vi "Math_2_Term_API_Hierarchy.vi"   [LabVIEW 2021]
uses:
  Support/Add/DBL/Add_DBL.lvclass
  Support/Subtract/DBL/Subtract_DBL.lvclass
  Support/Function/Two Terminal/SGL/AbsFunc_Two Term_SGL.lvclass
  Support/Function/Two Terminal/DBL/AbsFunc_Two Term_DBL.lvclass
  Support/Function/Two Terminal/EXT/AbsFunc_Two Term_EXT.lvclass
  Support/Function/Two Terminal/Cmplx SGL/AbsFunc_Two Term_Complex SGL.lvclass
  Support/Function/Two Terminal/Cmplx DBL/AbsFunc_Two Term_Complex DBL.lvclass
  Support/Function/Two Terminal/Cmplx EXT/AbsFunc_Two Term_Complex EXT.lvclass
  Support/Function/Two Terminal/I8/AbsFunc_Two Term_I8.lvclass
  Support/Function/Two Terminal/I16/AbsFunc_Two Term_I16.lvclass
  Support/Function/Two Terminal/I32/AbsFunc_Two Term_I32.lvclass
  Support/Function/Two Terminal/I64/AbsFunc_Two Term_I64.lvclass
  Support/Function/Two Terminal/U8/AbsFunc_Two Term_U8.lvclass
  Support/Function/Two Terminal/U16/AbsFunc_Two Term_U16.lvclass
  Support/Function/Two Terminal/U32/AbsFunc_Two Term_U32.lvclass
  Support/Function/Two Terminal/U64/AbsFunc_Two Term_U64.lvclass
  Support/Function/Two Terminal/WFM_Numeric/AbsFunc_Two Term_WFM_Numeric.lvclass
  Support/Function/Two Terminal/Time/AbsFunc_Two Term_Time.lvclass
  Support/Add/SGL/Add_SGL.lvclass
  Support/Add/EXT/Add_EXT.lvclass
  Support/Add/CPLX_SGL/Add_CPLX_SGL.lvclass
  Support/Add/CPLX_DBL/Add_CPLX_DBL.lvclass
  Support/Add/CPLX_EXT/Add_CPLX_EXT.lvclass
  Support/Add/I8/Add_I8.lvclass
  Support/Add/I16/Add_I16.lvclass
  Support/Add/I32/Add_I32.lvclass
  Support/Add/I64/Add_I64.lvclass
  Support/Add/U8/Add_U8.lvclass
  Support/Add/U16/Add_U16.lvclass
  Support/Add/U32/Add_U32.lvclass
  Support/Add/U64/Add_U64.lvclass
  Support/Add/Time/Add_Time.lvclass
  Support/Add/WFM_Numeric/Add_WFM_Numeric.lvclass
  Support/Subtract/SGL/Subtract_SGL.lvclass
  Support/Subtract/EXT/Subtract_EXT.lvclass
  Support/Subtract/CPLX_SGL/Subtract_CPLX_SGL.lvclass
  Support/Subtract/CPLX_DBL/Subtract_CPLX_DBL.lvclass
  Support/Subtract/CPLX_EXT/Subtract_CPLX_EXT.lvclass
  Support/Subtract/I8/Subtract_I8.lvclass
  Support/Subtract/I16/Subtract_I16.lvclass
  Support/Subtract/I32/Subtract_I32.lvclass
  Support/Subtract/I64/Subtract_I64.lvclass
  Support/Subtract/U8/Subtract_U8.lvclass
  Support/Subtract/U16/Subtract_U16.lvclass
  Support/Subtract/U32/Subtract_U32.lvclass
  Support/Subtract/U64/Subtract_U64.lvclass
  Support/Subtract/Time/Subtract_Time.lvclass
  Support/Multiply/DBL/Multiply_DBL.lvclass
  Support/Subtract/WFM_Numeric/Subtract_WFM_Numeric.lvclass
  Support/Multiply/SGL/Multiply_SGL.lvclass
  Support/Multiply/EXT/Multiply_EXT.lvclass
  Support/Multiply/CPLX_SGL/Multiply_CPLX_SGL.lvclass
  Support/Multiply/CPLX_DBL/Multiply_CPLX_DBL.lvclass
  Support/Multiply/CPLX_EXT/Multiply_CPLX_EXT.lvclass
  Support/Multiply/I8/Multiply_I8.lvclass
  Support/Multiply/I16/Multiply_I16.lvclass
  Support/Multiply/I32/Multiply_I32.lvclass
  Support/Multiply/I64/Multiply_I64.lvclass
  Support/Multiply/U8/Multiply_U8.lvclass
  Support/Multiply/U16/Multiply_U16.lvclass
  Support/Multiply/U32/Multiply_U32.lvclass
  Support/Multiply/U64/Multiply_U64.lvclass
  Support/Multiply/WFM_Numeric/Multiply_WFM_Numeric.lvclass
  Support/Divide/SGL/Divide_SGL.lvclass
  Support/Divide/DBL/Divide_DBL.lvclass
  Support/Divide/EXT/Divide_EXT.lvclass
  Support/Divide/CPLX_DBL/Divide_CPLX_DBL.lvclass
  Support/Divide/CPLX_EXT/Divide_CPLX_EXT.lvclass
  Support/Divide/CPLX_SGL/Divide_CPLX_SGL.lvclass
  Support/Divide/WFM_Numeric/Divide_WFM_Numeric.lvclass
  Support/Subtract/Time-Time/Subtract_Time-Time.lvclass
  Abs_Types/Double Float/Abs_Double Float.lvclass
  Support/Divide/INT/Divide_INT.lvclass
panel:
  # "SEE DIAGRAM\nFOR Hierarchy"
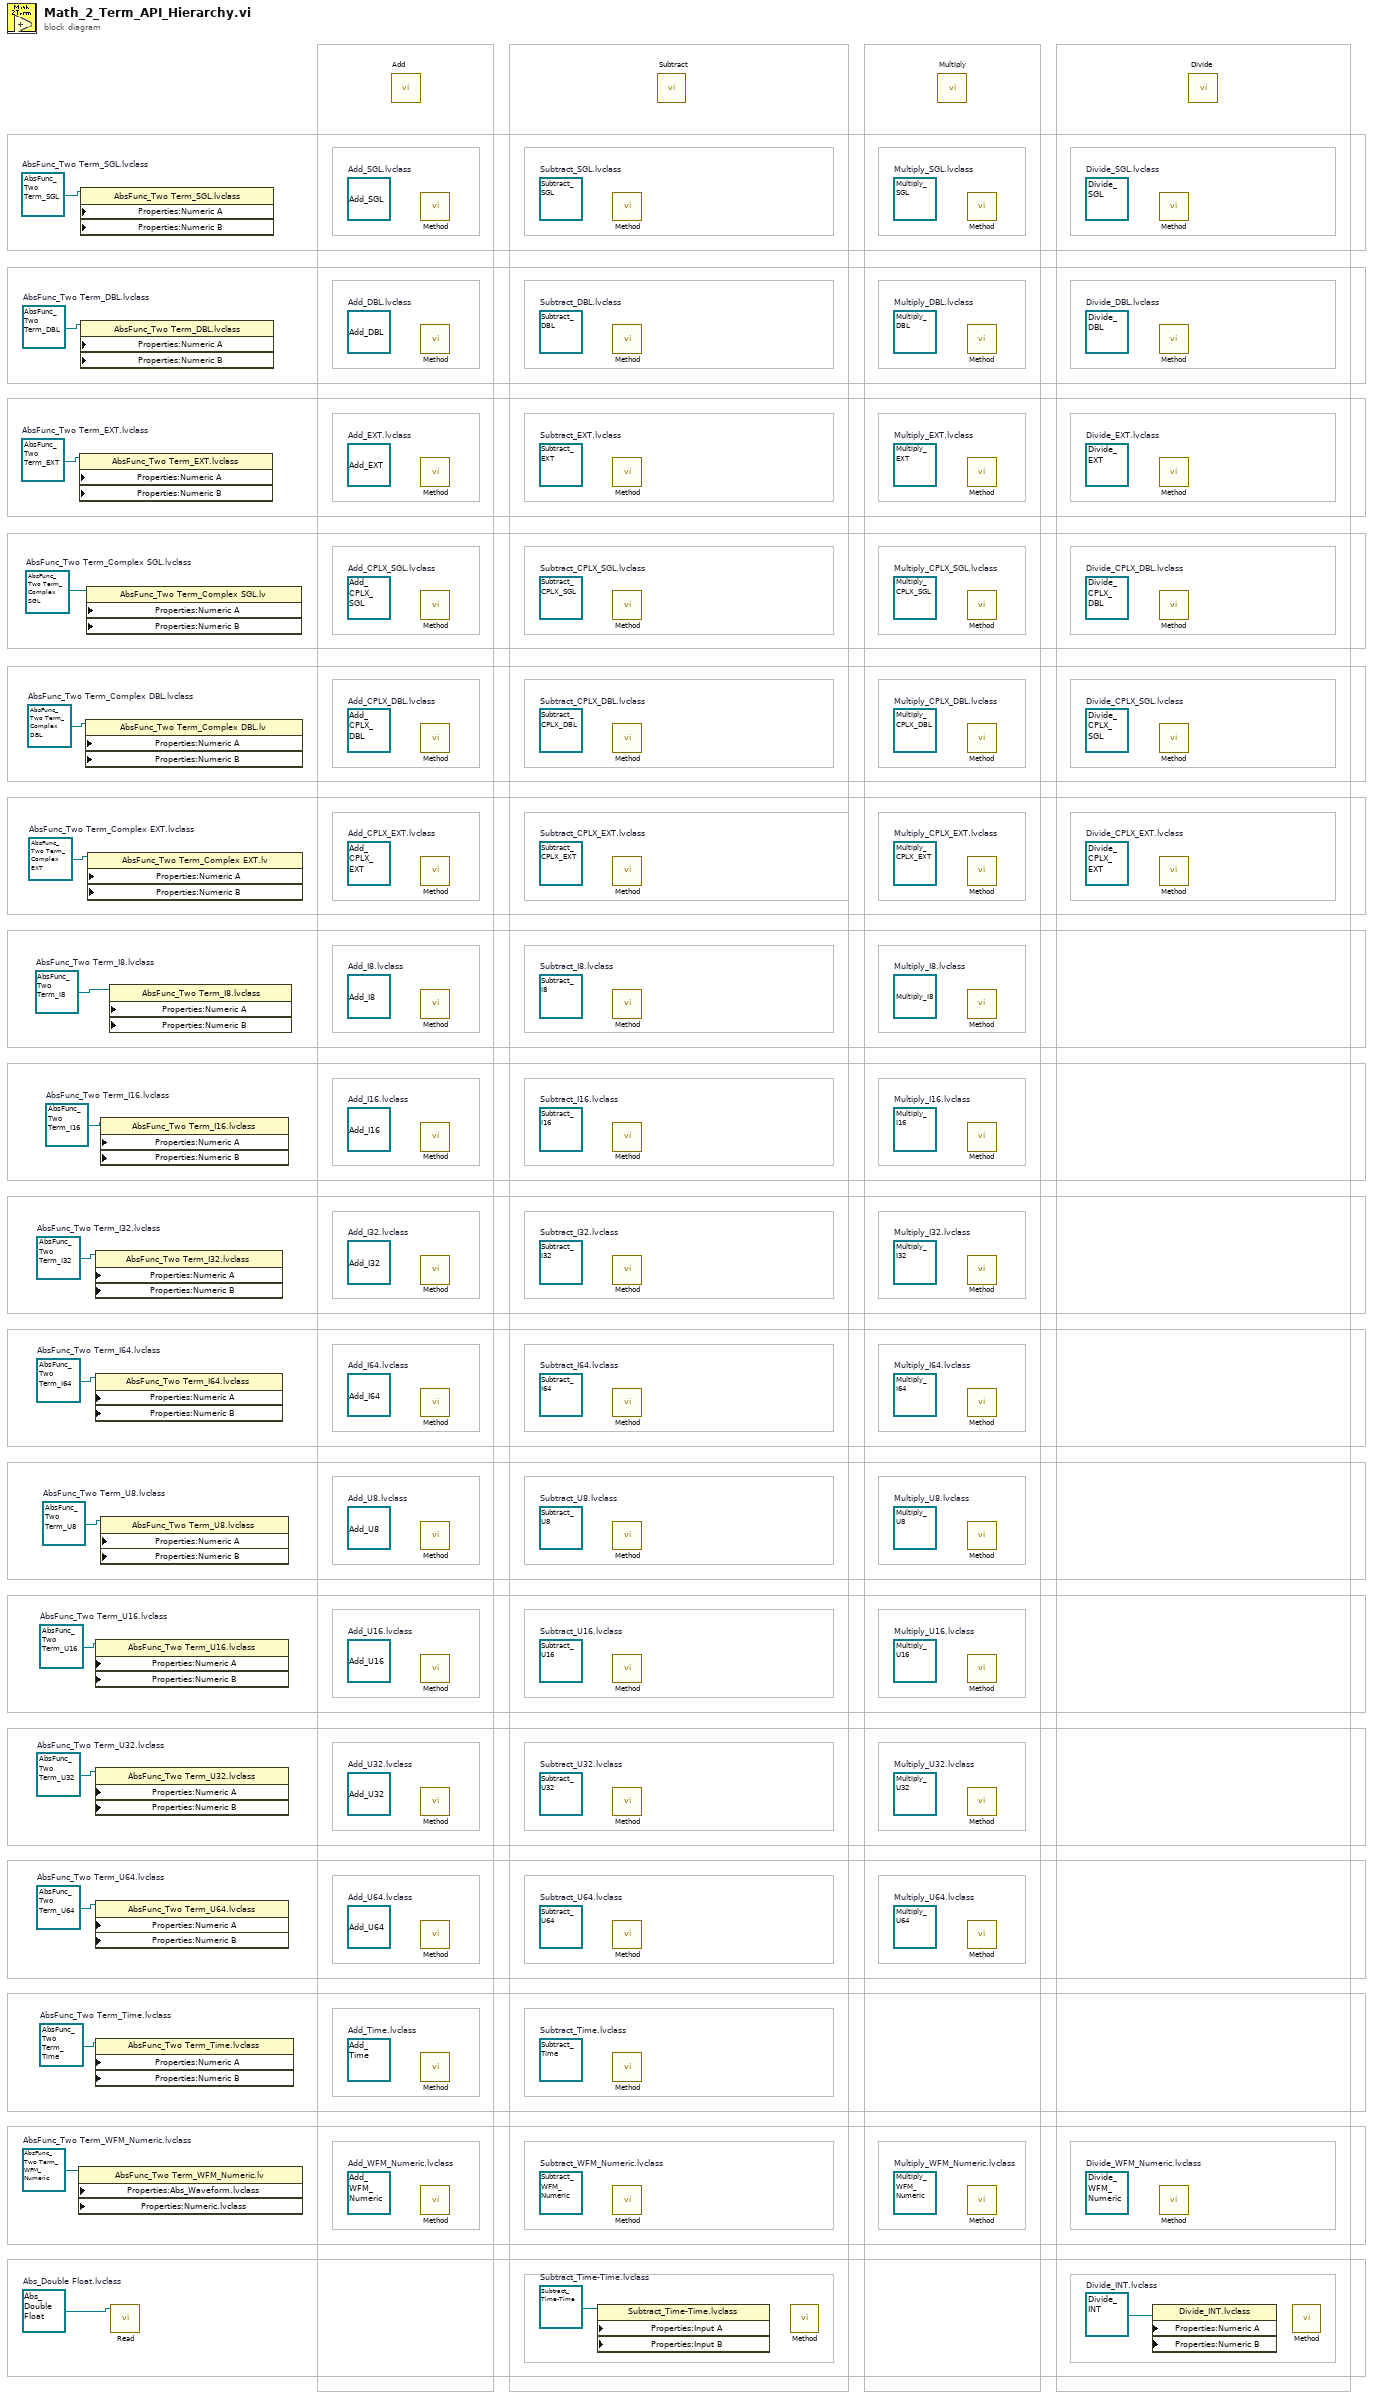
[diagram p0: block diagram]
diagram:
  w1 = refnum<class "Divide_INT.lvclass"> refnum  # Divide_INT.lvclass
  w2 = refnum<class "Abs_Double Float.lvclass"> refnum  # Abs_Double Float.lvclass
  w3 = refnum<class "Subtract_Time-Time.lvclass"> refnum  # Subtract_Time-Time.lvclass
  (unwired) refnum<class "Divide_WFM_Numeric.lvclass"> refnum  # Divide_WFM_Numeric.lvclass
  (unwired) refnum<class "Divide_CPLX_SGL.lvclass"> refnum  # Divide_CPLX_SGL.lvclass
  (unwired) refnum<class "Divide_CPLX_EXT.lvclass"> refnum  # Divide_CPLX_EXT.lvclass
  (unwired) refnum<class "Divide_CPLX_DBL.lvclass"> refnum  # Divide_CPLX_DBL.lvclass
  (unwired) refnum<class "Divide_EXT.lvclass"> refnum  # Divide_EXT.lvclass
  (unwired) refnum<class "Divide_DBL.lvclass"> refnum  # Divide_DBL.lvclass
  (unwired) refnum<class "Divide_SGL.lvclass"> refnum  # Divide_SGL.lvclass
  (unwired) refnum<class "Multiply_WFM_Numeric.lvclass"> refnum  # Multiply_WFM_Numeric.lvclass
  (unwired) refnum<class "Multiply_U64.lvclass"> refnum  # Multiply_U64.lvclass
  (unwired) refnum<class "Multiply_U32.lvclass"> refnum  # Multiply_U32.lvclass
  (unwired) refnum<class "Multiply_U16.lvclass"> refnum  # Multiply_U16.lvclass
  (unwired) refnum<class "Multiply_U8.lvclass"> refnum  # Multiply_U8.lvclass
  (unwired) refnum<class "Multiply_I64.lvclass"> refnum  # Multiply_I64.lvclass
  (unwired) refnum<class "Multiply_I32.lvclass"> refnum  # Multiply_I32.lvclass
  (unwired) refnum<class "Multiply_I16.lvclass"> refnum  # Multiply_I16.lvclass
  (unwired) refnum<class "Multiply_I8.lvclass"> refnum  # Multiply_I8.lvclass
  (unwired) refnum<class "Multiply_CPLX_EXT.lvclass"> refnum  # Multiply_CPLX_EXT.lvclass
  (unwired) refnum<class "Multiply_CPLX_DBL.lvclass"> refnum  # Multiply_CPLX_DBL.lvclass
  (unwired) refnum<class "Multiply_CPLX_SGL.lvclass"> refnum  # Multiply_CPLX_SGL.lvclass
  (unwired) refnum<class "Multiply_EXT.lvclass"> refnum  # Multiply_EXT.lvclass
  (unwired) refnum<class "Multiply_DBL.lvclass"> refnum  # Multiply_DBL.lvclass
  (unwired) refnum<class "Multiply_SGL.lvclass"> refnum  # Multiply_SGL.lvclass
  (unwired) refnum<class "Subtract_WFM_Numeric.lvclass"> refnum  # Subtract_WFM_Numeric.lvclass
  (unwired) refnum<class "Subtract_Time.lvclass"> refnum  # Subtract_Time.lvclass
  (unwired) refnum<class "Subtract_U64.lvclass"> refnum  # Subtract_U64.lvclass
  (unwired) refnum<class "Subtract_U32.lvclass"> refnum  # Subtract_U32.lvclass
  (unwired) refnum<class "Subtract_U16.lvclass"> refnum  # Subtract_U16.lvclass
  (unwired) refnum<class "Subtract_U8.lvclass"> refnum  # Subtract_U8.lvclass
  (unwired) refnum<class "Subtract_I64.lvclass"> refnum  # Subtract_I64.lvclass
  (unwired) refnum<class "Subtract_I32.lvclass"> refnum  # Subtract_I32.lvclass
  (unwired) refnum<class "Subtract_I16.lvclass"> refnum  # Subtract_I16.lvclass
  (unwired) refnum<class "Subtract_I8.lvclass"> refnum  # Subtract_I8.lvclass
  (unwired) refnum<class "Subtract_CPLX_EXT.lvclass"> refnum  # Subtract_CPLX_EXT.lvclass
  (unwired) refnum<class "Subtract_CPLX_DBL.lvclass"> refnum  # Subtract_CPLX_DBL.lvclass
  (unwired) refnum<class "Subtract_CPLX_SGL.lvclass"> refnum  # Subtract_CPLX_SGL.lvclass
  (unwired) refnum<class "Subtract_EXT.lvclass"> refnum  # Subtract_EXT.lvclass
  (unwired) refnum<class "Subtract_DBL.lvclass"> refnum  # Subtract_DBL.lvclass
  (unwired) refnum<class "Subtract_SGL.lvclass"> refnum  # Subtract_SGL.lvclass
  (unwired) refnum<class "Add_WFM_Numeric.lvclass"> refnum  # Add_WFM_Numeric.lvclass
  (unwired) refnum<class "Add_Time.lvclass"> refnum  # Add_Time.lvclass
  (unwired) refnum<class "Add_U64.lvclass"> refnum  # Add_U64.lvclass
  (unwired) refnum<class "Add_U32.lvclass"> refnum  # Add_U32.lvclass
  (unwired) refnum<class "Add_U16.lvclass"> refnum  # Add_U16.lvclass
  (unwired) refnum<class "Add_U8.lvclass"> refnum  # Add_U8.lvclass
  (unwired) refnum<class "Add_I64.lvclass"> refnum  # Add_I64.lvclass
  (unwired) refnum<class "Add_I32.lvclass"> refnum  # Add_I32.lvclass
  (unwired) refnum<class "Add_I16.lvclass"> refnum  # Add_I16.lvclass
  (unwired) refnum<class "Add_I8.lvclass"> refnum  # Add_I8.lvclass
  (unwired) refnum<class "Add_CPLX_EXT.lvclass"> refnum  # Add_CPLX_EXT.lvclass
  (unwired) refnum<class "Add_CPLX_DBL.lvclass"> refnum  # Add_CPLX_DBL.lvclass
  (unwired) refnum<class "Add_CPLX_SGL.lvclass"> refnum  # Add_CPLX_SGL.lvclass
  (unwired) refnum<class "Add_EXT.lvclass"> refnum  # Add_EXT.lvclass
  (unwired) refnum<class "Add_SGL.lvclass"> refnum  # Add_SGL.lvclass
  (unwired) refnum<class "Add_DBL.lvclass"> refnum  # Add_DBL.lvclass
  w4 = refnum<class "AbsFunc_Two Term_Time.lvclass"> refnum  # AbsFunc_Two Term_Time.lvclass
  w5 = refnum<class "AbsFunc_Two Term_WFM_Numeric.lvclass"> refnum  # AbsFunc_Two Term_WFM_Numeric.lvclass
  w6 = refnum<class "AbsFunc_Two Term_U64.lvclass"> refnum  # AbsFunc_Two Term_U64.lvclass
  w7 = refnum<class "AbsFunc_Two Term_U32.lvclass"> refnum  # AbsFunc_Two Term_U32.lvclass
  w8 = refnum<class "AbsFunc_Two Term_U16.lvclass"> refnum  # AbsFunc_Two Term_U16.lvclass
  w9 = refnum<class "AbsFunc_Two Term_U8.lvclass"> refnum  # AbsFunc_Two Term_U8.lvclass
  w10 = refnum<class "AbsFunc_Two Term_I64.lvclass"> refnum  # AbsFunc_Two Term_I64.lvclass
  w11 = refnum<class "AbsFunc_Two Term_I32.lvclass"> refnum  # AbsFunc_Two Term_I32.lvclass
  w12 = refnum<class "AbsFunc_Two Term_I16.lvclass"> refnum  # AbsFunc_Two Term_I16.lvclass
  w13 = refnum<class "AbsFunc_Two Term_I8.lvclass"> refnum  # AbsFunc_Two Term_I8.lvclass
  w14 = refnum<class "AbsFunc_Two Term_Complex EXT.lvclass"> refnum  # AbsFunc_Two Term_Complex EXT.lvclass
  w15 = refnum<class "AbsFunc_Two Term_Complex DBL.lvclass"> refnum  # AbsFunc_Two Term_Complex DBL.lvclass
  w16 = refnum<class "AbsFunc_Two Term_Complex SGL.lvclass"> refnum  # AbsFunc_Two Term_Complex SGL.lvclass
  w17 = refnum<class "AbsFunc_Two Term_EXT.lvclass"> refnum  # AbsFunc_Two Term_EXT.lvclass
  w18 = refnum<class "AbsFunc_Two Term_DBL.lvclass"> refnum  # AbsFunc_Two Term_DBL.lvclass
  w19 = refnum<class "AbsFunc_Two Term_SGL.lvclass"> refnum  # AbsFunc_Two Term_SGL.lvclass
  n1 = property class="AbsFunc_Two Term_WFM_Numeric.lv" props=["Properties:Abs_Waveform.lvclass", "Properties:Numeric.lvclass"](reference=w5) -> ()  [unwired: 3 in, 2 out]
  n2 = property class="AbsFunc_Two Term_EXT.lvclass" props=["Properties:Numeric A", "Properties:Numeric B"](reference=w17) -> ()  [unwired: 3 in, 2 out]
  n3 = property class="AbsFunc_Two Term_SGL.lvclass" props=["Properties:Numeric A", "Properties:Numeric B"](reference=w19) -> ()  [unwired: 3 in, 2 out]
  n4 = property class="AbsFunc_Two Term_DBL.lvclass" props=["Properties:Numeric A", "Properties:Numeric B"](reference=w18) -> ()  [unwired: 3 in, 2 out]
  n5 = property class="AbsFunc_Two Term_Complex DBL.lv" props=["Properties:Numeric A", "Properties:Numeric B"](reference=w15) -> ()  [unwired: 3 in, 2 out]
  n6 = property class="AbsFunc_Two Term_Complex SGL.lv" props=["Properties:Numeric A", "Properties:Numeric B"](reference=w16) -> ()  [unwired: 3 in, 2 out]
  n7 = property class="AbsFunc_Two Term_Complex EXT.lv" props=["Properties:Numeric A", "Properties:Numeric B"](reference=w14) -> ()  [unwired: 3 in, 2 out]
  n8 = property class="AbsFunc_Two Term_I32.lvclass" props=["Properties:Numeric A", "Properties:Numeric B"](reference=w11) -> ()  [unwired: 3 in, 2 out]
  n9 = property class="AbsFunc_Two Term_I64.lvclass" props=["Properties:Numeric A", "Properties:Numeric B"](reference=w10) -> ()  [unwired: 3 in, 2 out]
  n10 = property class="AbsFunc_Two Term_U16.lvclass" props=["Properties:Numeric A", "Properties:Numeric B"](reference=w8) -> ()  [unwired: 3 in, 2 out]
  n11 = property class="AbsFunc_Two Term_U32.lvclass" props=["Properties:Numeric A", "Properties:Numeric B"](reference=w7) -> ()  [unwired: 3 in, 2 out]
  n12 = property class="AbsFunc_Two Term_U64.lvclass" props=["Properties:Numeric A", "Properties:Numeric B"](reference=w6) -> ()  [unwired: 3 in, 2 out]
  n13 = property class="AbsFunc_Two Term_Time.lvclass" props=["Properties:Numeric A", "Properties:Numeric B"](reference=w4) -> ()  [unwired: 3 in, 2 out]
  n14 = property class="AbsFunc_Two Term_I16.lvclass" props=["Properties:Numeric A", "Properties:Numeric B"](reference=w12) -> ()  [unwired: 3 in, 2 out]
  n15 = property class="AbsFunc_Two Term_U8.lvclass" props=["Properties:Numeric A", "Properties:Numeric B"](reference=w9) -> ()  [unwired: 3 in, 2 out]
  n16 = property class="AbsFunc_Two Term_I8.lvclass" props=["Properties:Numeric A", "Properties:Numeric B"](reference=w13) -> ()  [unwired: 3 in, 2 out]
  n17 = call-dynamic "Read.vi"("Double Float.lvclass_340760 in"=w2) -> ()  [unwired: 8 in, 3 out]
  n18 = call-poly "Add.vi"() -> ()  [unwired: 6 in, 1 out]
  n19 = call "Method.vi"() -> ()  [unwired: 6 in, 1 out]
  n20 = call "Method.vi"() -> ()  [unwired: 6 in, 1 out]
  n21 = call "Method.vi"() -> ()  [unwired: 6 in, 1 out]
  n22 = call "Method.vi"() -> ()  [unwired: 6 in, 1 out]
  n23 = call "Method.vi"() -> ()  [unwired: 6 in, 1 out]
  n24 = call "Method.vi"() -> ()  [unwired: 6 in, 1 out]
  n25 = call "Method.vi"() -> ()  [unwired: 6 in, 1 out]
  n26 = call "Method.vi"() -> ()  [unwired: 6 in, 1 out]
  n27 = call "Method.vi"() -> ()  [unwired: 6 in, 1 out]
  n28 = call "Method.vi"() -> ()  [unwired: 6 in, 1 out]
  n29 = call "Method.vi"() -> ()  [unwired: 6 in, 1 out]
  n30 = call "Method.vi"() -> ()  [unwired: 6 in, 1 out]
  n31 = call "Method.vi"() -> ()  [unwired: 6 in, 1 out]
  n32 = call "Method.vi"() -> ()  [unwired: 6 in, 1 out]
  n33 = call "Method.vi"() -> ()  [unwired: 6 in, 1 out]
  n34 = call "Method.vi"() -> ()  [unwired: 6 in, 1 out]
  n35 = property class="Subtract_Time-Time.lvclass" props=["Properties:Input A", "Properties:Input B"](reference=w3) -> ()  [unwired: 3 in, 2 out]
  n36 = call "Method.vi"() -> ()  [unwired: 6 in, 1 out]
  n37 = call "Method.vi"() -> ()  [unwired: 6 in, 1 out]
  n38 = call "Method.vi"() -> ()  [unwired: 6 in, 1 out]
  n39 = call "Method.vi"() -> ()  [unwired: 6 in, 1 out]
  n40 = call "Method.vi"() -> ()  [unwired: 6 in, 1 out]
  n41 = call "Method.vi"() -> ()  [unwired: 6 in, 1 out]
  n42 = call "Method.vi"() -> ()  [unwired: 6 in, 1 out]
  n43 = call "Method.vi"() -> ()  [unwired: 6 in, 1 out]
  n44 = call "Method.vi"() -> ()  [unwired: 6 in, 1 out]
  n45 = call "Method.vi"() -> ()  [unwired: 6 in, 1 out]
  n46 = call "Method.vi"() -> ()  [unwired: 6 in, 1 out]
  n47 = call "Method.vi"() -> ()  [unwired: 6 in, 1 out]
  n48 = call "Method.vi"() -> ()  [unwired: 6 in, 1 out]
  n49 = call "Method.vi"() -> ()  [unwired: 6 in, 1 out]
  n50 = call "Method.vi"() -> ()  [unwired: 6 in, 1 out]
  n51 = call "Method.vi"() -> ()  [unwired: 6 in, 1 out]
  n52 = call-poly "Subtract.vi"() -> ()  [unwired: 6 in, 1 out]
  n53 = call "Method.vi"() -> ()  [unwired: 6 in, 1 out]
  n54 = call-poly "Multiply.vi"() -> ()  [unwired: 6 in, 1 out]
  n55 = call "Method.vi"() -> ()  [unwired: 6 in, 1 out]
  n56 = call "Method.vi"() -> ()  [unwired: 6 in, 1 out]
  n57 = call "Method.vi"() -> ()  [unwired: 6 in, 1 out]
  n58 = call "Method.vi"() -> ()  [unwired: 6 in, 1 out]
  n59 = call "Method.vi"() -> ()  [unwired: 6 in, 1 out]
  n60 = call "Method.vi"() -> ()  [unwired: 6 in, 1 out]
  n61 = call "Method.vi"() -> ()  [unwired: 6 in, 1 out]
  n62 = call "Method.vi"() -> ()  [unwired: 6 in, 1 out]
  n63 = call "Method.vi"() -> ()  [unwired: 6 in, 1 out]
  n64 = call "Method.vi"() -> ()  [unwired: 6 in, 1 out]
  n65 = call "Method.vi"() -> ()  [unwired: 6 in, 1 out]
  n66 = call "Method.vi"() -> ()  [unwired: 6 in, 1 out]
  n67 = call "Method.vi"() -> ()  [unwired: 6 in, 1 out]
  n68 = call "Method.vi"() -> ()  [unwired: 6 in, 1 out]
  n69 = call "Method.vi"() -> ()  [unwired: 6 in, 1 out]
  n70 = property class="Divide_INT.lvclass" props=["Properties:Numeric A", "Properties:Numeric B"](reference=w1) -> ()  [unwired: 3 in, 2 out]
  n71 = call "Method.vi"() -> ()  [unwired: 6 in, 1 out]
  n72 = call "Method.vi"() -> ()  [unwired: 6 in, 1 out]
  n73 = call "Method.vi"() -> ()  [unwired: 6 in, 1 out]
  n74 = call "Method.vi"() -> ()  [unwired: 6 in, 1 out]
  n75 = call "Method.vi"() -> ()  [unwired: 6 in, 1 out]
  n76 = call "Method.vi"() -> ()  [unwired: 6 in, 1 out]
  n77 = call "Method.vi"() -> ()  [unwired: 6 in, 1 out]
  n78 = call-poly "Divide.vi"() -> ()  [unwired: 6 in, 1 out]
  n79 = call "Method.vi"() -> ()  [unwired: 6 in, 1 out]
